vi "DAQ_general.vi"() -> ()   [LabVIEW 2024]
panel:
  in  "milliseconds to wait":u32
  out "element":u32
  in  "IP LABVIEW":string="192.168.1.26"
  in  "PUERTO LABVIEW":i32=8000
  in  "PUERTO ENVIO":i32=8001
  in  "IP ENVIO":string="192.168.1.52"
  in  "STOP ENVIO":bool
  out "error out 4":errorcluster
  in  "ENVIO DE DATOS":u8[](array[numeric])
  out "Boolean":bool
  out "element 9":bool
  out "element 8":bool
  out "element 7":bool
  out "element 6":bool
  out "Waveform Chart 4":waveform(dbl)(graph)
  out "Waveform Chart 3":waveform(dbl)(graph)
  out "DIG 4 DIG 4":bool
  out "DIG 3":bool
  out "DIG 2":bool
  out "DIG1":bool
  out "ANALOGICO 2 Chart 2":waveform(dbl)(graph)
  out "ANALOGICO 1 Chart":waveform(dbl)(graph)
  out "error out 3":errorcluster
  in  "STOP RECEPCION":bool
  out "ANALOGICO 2":u16[](array[numeric])
  out "ANALOGICO 1":u16[](array[numeric])
  out "error out 2":errorcluster
  in  "STOP BUCLE PRINCIAL":bool
  out "error out":errorcluster
  out "connection ID":refnum<k16>
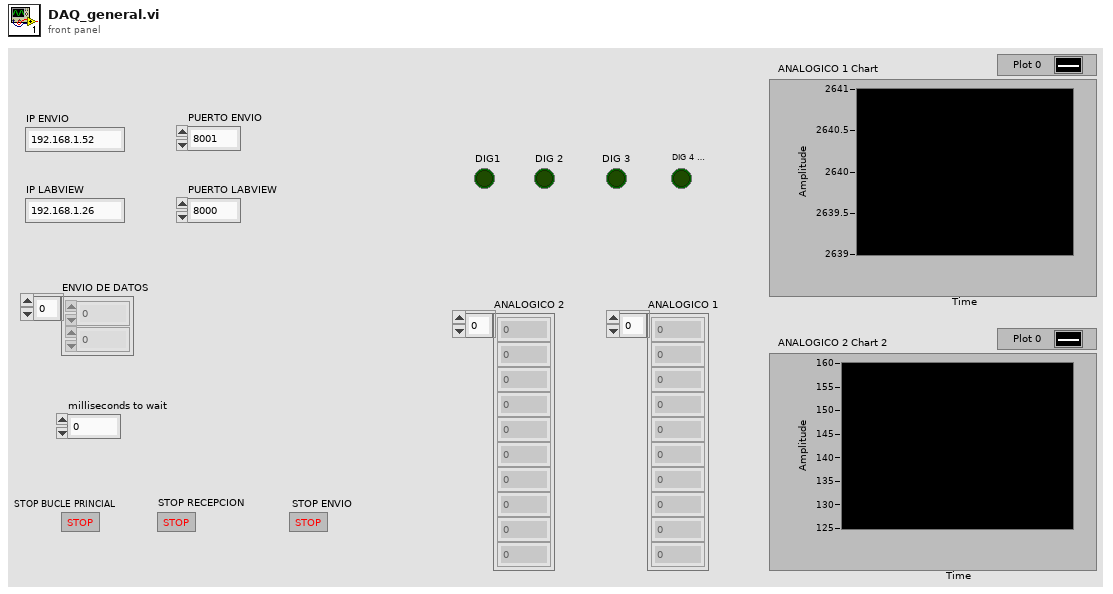
[diagram p1: front panel]
types:
  T1 = enum16{"big-endian, network order", "native, host order", "little-endian"}
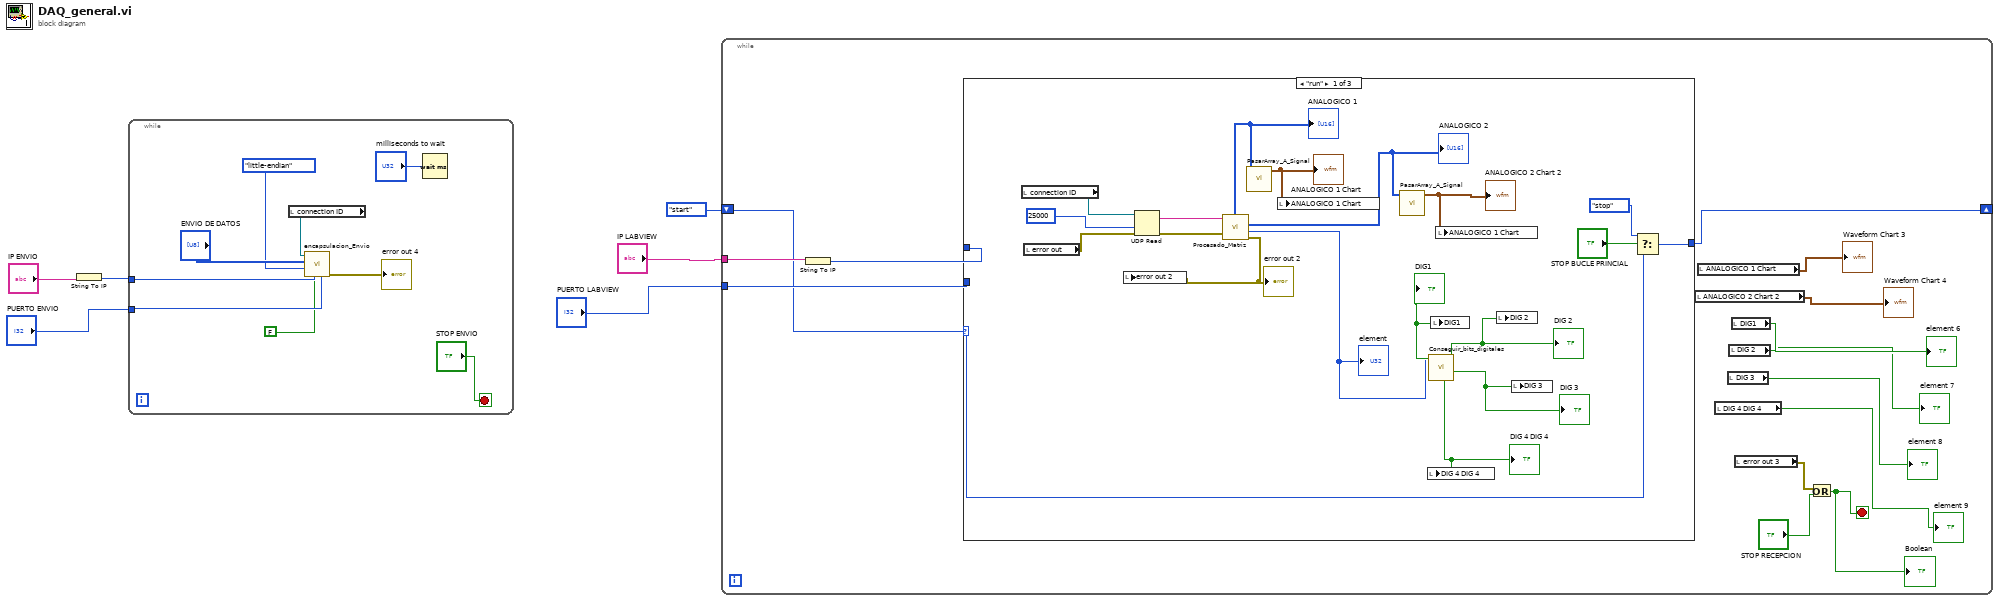
[diagram p0: block diagram]
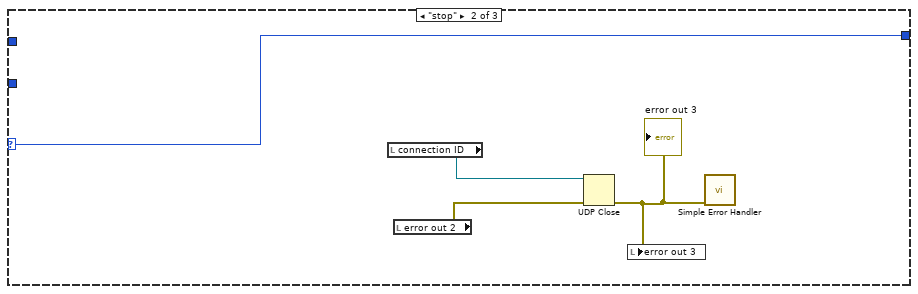
[diagram p2: hidden frame]
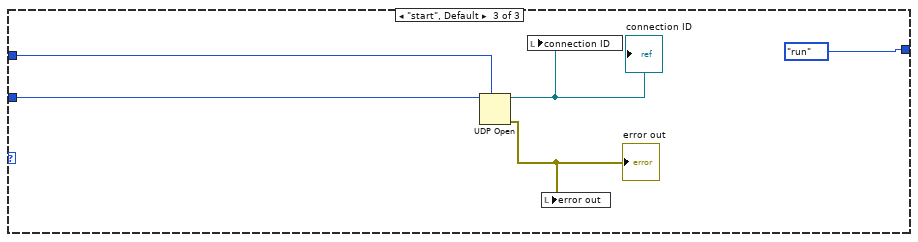
[diagram p3: hidden frame]
diagram:
  n1 = String To IP(1:"IP ENVIO") -> (0:w5:u32)
  n2 = while {
    tunnel: "PUERTO ENVIO" -> [w14]
    tunnel: w5 -> [w13]
    stop <- "STOP ENVIO" stop-if-true
    n3 = local read "connection ID"() -> (w15:refnum<k16>)
    n4 = call "encapsulacion_Envio.vi"("PORT"=w14, "prepend array or string size? (T)"=FALSE, "Numeric 2"=w13, "byte order (0:big-endian, network order)"=T1."little-endian", "Array"="ENVIO DE DATOS", "UDP Network Connection in"=w15) -> ("error out"=→"error out 4":errorcluster)  [unwired: 5 in]
    n5 = Wait (ms)(milliseconds to wait="milliseconds to wait") -> ()  [unwired: 1 out]
  }
  n6 = while {
    tunnel: "IP LABVIEW" -> [w29]
    tunnel: "PUERTO LABVIEW" -> [w27]
    shift-right: [w26] -> _
    shift-left: enum16{"", "start", "run", "stop"}."start" -> [w25]
    stop <- w22 stop-if-true
    n7 = String To IP(1:w29) -> (0:w28:u32)
    n8 = case shown="\"run\"" w25 {
      selector: w25 -> [w41 w50 _]
      tunnel: w28 -> [_ _ w57]
      tunnel: w27 -> [_ _ w56]
      tunnel: [w45 w50 enum16{"", "start", "run", "stop"}."run"] -> w26
      frame "run" {
        n9 = local read "connection ID"() -> (w48:refnum<k16>)
        n10 = local read "error out"() -> (w32:errorcluster)
        n11 = UDP Read(connection ID=w48, timeout ms (25000)=25000, 8:w32) -> (data out=w44:string, error out=w43:errorcluster)  [unwired: 1 in, 3 out]
        n12 = call "Procesado_Matriz.vi"("error in (no error)"=w43, "data in"=w44) -> ("error out"=w42:errorcluster, "element"=w30:u32, "subarray 2"=w39:u16[], "subarray"=w40:u16[])  [unwired: 6 in]
        "error out 2" <- w42
        "ANALOGICO 1" <- w40
        "ANALOGICO 2" <- w39
        "element" <- w30
        n13 = local write "error out 2"(w42) -> ()
        n14 = call "PasarArray_A_Signal.vi"("subarray"=w40) -> ("Waveform"=w33:waveform(dbl))  [unwired: 10 in]
        "ANALOGICO 1 Chart" <- w33
        n15 = local write "ANALOGICO 1 Chart"(w33) -> ()
        n16 = call "PasarArray_A_Signal.vi"("subarray"=w39) -> ("Waveform"=w34:waveform(dbl))  [unwired: 10 in]
        "ANALOGICO 2 Chart 2" <- w34
        n17 = call "Conseguir_bits_digitales.vi"("element"=w30) -> ("Boolean 2"=w37:bool, "Boolean 3"=w36:bool, "Boolean 4"=w35:bool, "Boolean"=w38:bool)  [unwired: 7 in]
        "DIG1" <- w35
        "DIG 2" <- w36
        "DIG 3" <- w37
        "DIG 4 DIG 4" <- w38
        n18 = local write "DIG 4 DIG 4"(w38) -> ()
        n19 = local write "DIG1"(w35) -> ()
        n20 = local write "ANALOGICO 1 Chart"(w34) -> ()
        n21 = local write "DIG 2"(w36) -> ()
        n22 = local write "DIG 3"(w37) -> ()
        n23 = Select(t=enum16{"", "start", "run", "stop"}."stop", s="STOP BUCLE PRINCIAL", f=w41) -> (s? t:f=w45:enum16{"", "start", "run", "stop"})
      }
      frame "stop" {
        n24 = local read "connection ID"() -> (w52:refnum<k16>)
        n25 = local read "error out 2"() -> (w51:errorcluster)
        n26 = UDP Close(connection ID=w52, 8:w51) -> (error out=w49:errorcluster)  [unwired: 1 out]
        "error out 3" <- w49
        n27 = local write "error out 3"(w49) -> ()
        n28 = call <vilib>:"Simple Error Handler.vi"("error in (no error)"=w49) -> ()  [unwired: 4 in, 5 out]
      }
      frame "start", Default {
        n29 = UDP Open(7:w57, 11:w56) -> (port=w53:refnum<k16>, 0:w55:errorcluster)  [unwired: 3 in, 1 out]
        "connection ID" <- w53
        "error out" <- w55
        n30 = local write "connection ID"(w53) -> ()
        n31 = local write "error out"(w55) -> ()
      }
    }
    n32 = local read "ANALOGICO 2 Chart 2"() -> (→"Waveform Chart 4":waveform(dbl))
    n33 = local read "ANALOGICO 1 Chart"() -> (→"Waveform Chart 3":waveform(dbl))
    n34 = local read "DIG 4 DIG 4"() -> (→"element 9":bool)
    n35 = local read "DIG 3"() -> (→"element 8":bool)
    n36 = local read "DIG 2"() -> (→"element 7":bool)
    n37 = local read "DIG1"() -> (→"element 6":bool)
    n38 = local read "error out 3"() -> (w23:errorcluster)
    n39 = Or(x=w23, y="STOP RECEPCION") -> (x .or. y?=w22:bool)
    "Boolean" <- w22
  }
